vi "Broadcast Shutter State.vi"(8 "error in (no error)":errorcluster, 10 "Reply Payload":T1={"Shutter State"=enum."Open", "Set Shutter State_error"={"status"=FALSE, "code"=0, "source"=""}}) -> (0 "error out":errorcluster)   [LabVIEW 2020, in "Shutter.lvlib"]
doc: "_____\nCreated using Delacor QMH Event Scripter 5.0.0.112."
uses:
  Shutter.lvlib
  Set Shutter State (Reply Payload)--cluster.ctl
  Shutter State.ctl
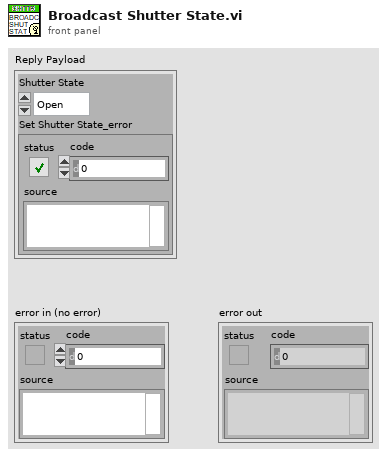
[diagram p1: front panel]
types:
  T1 = typedef "Shutter.lvlib/Set Shutter State (Reply Payload)--cluster.ctl" = cluster{"Shutter State":T2, "Set Shutter State_error":errorcluster}
  T2 = typedef "Shutter State.ctl" = enum16{"None", "Open", "Closed"}
  T3 = typedef "Shutter.lvlib/Broadcast Events--cluster.ctl" = cluster{"Module Did Init":refnum<user-event>, "Status Updated":refnum<user-event>, "Error Reported":refnum<user-event>, "Module Did Stop":refnum<user-event>, "Update Module Execution Status":refnum<user-event>, "Broadcast Shutter State":refnum<user-event>}
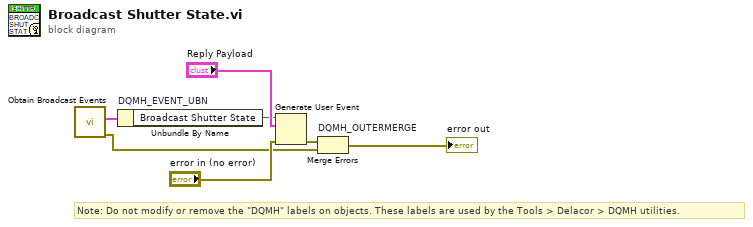
[diagram p0: block diagram]
diagram:
  # "Note: Do not modify or remove the \"DQMH\" labels on objects. These labels are used by the Tools > Delacor > DQMH utilities."
  n1 = call "Obtain Broadcast Events.vi"() -> ("error out"=w2:errorcluster, "Shutter Broadcast Events"=w1:T3)  [unwired: 10 in]
  n2 = Unbundle By Name "DQMH_EVENT_UBN"(w1) -> ("Broadcast Shutter State"=w4:refnum<user-event>)
  n3 = Generate User Event(user event=w4, event data cluster="Reply Payload", error in="error in (no error)") -> (error out=w3:errorcluster)  [unwired: 1 in, 1 out]
  n4 = Merge Errors "DQMH_OUTERMERGE"(w3, w2) -> (→"error out":errorcluster)
